vi "Labview8_3 (SubVI).vi"(6 "Input 4":dbl, 9 "Input 3":dbl, 10 "Input in":dbl, 11 "Input 1":dbl) -> (3 "Numeric":dbl)   [LabVIEW 2016]
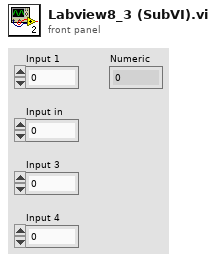
[diagram p1: front panel]
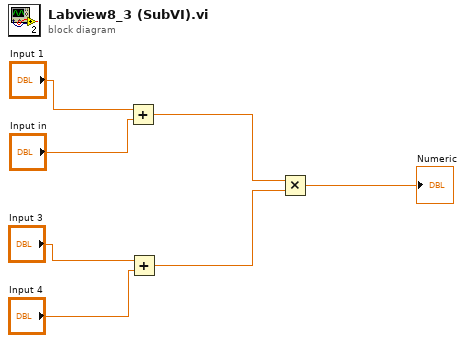
[diagram p0: block diagram]
diagram:
  n1 = Add(x="Input 1", y="Input in") -> (x+y=w5:dbl)
  n2 = Add(x="Input 3", y="Input 4") -> (x+y=w6:dbl)
  n3 = Multiply(x=w5, y=w6) -> (x*y=→"Numeric":dbl)
